vi "Clean errors.vi"(8 "error in (no error)":errorcluster) -> (0 "error out":errorcluster)   [LabVIEW 2020, in "Error Handler.lvlib"]
uses:
  Error Handler.lvlib
  Error Hander Def.ctl
  Def/Queue_Function Def.ctl
  Def/Queue_Method Def.ctl
  Def/Queue_Def.ctl
  <vilib>/MultiError/TokenizeJSON/Multi Error Cluster.lvlib
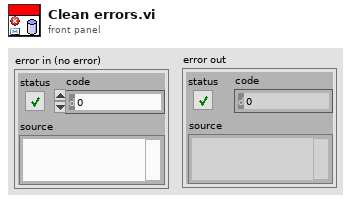
[diagram p1: front panel]
types:
  T1 = typedef "Queue_Def.ctl" = cluster{"Message":string, "Data":variant}
  T2 = typedef "Queue_Method Def.ctl" = enum16{"Initialize", "Read", "Write", "Insert", "Get_Specific_Quene_Status", "Flush Speciffic Quene", "Release All Quenes"}
  T3 = typedef "Queue_Function Def.ctl" = enum16{"MHL", "Return(Watch dog)", "Event Log", "Error Log"}
  T4 = typedef "Error Handler.lvlib/Error Hander Def.ctl" = cluster{"Time":timestamp, "Data":errorcluster}
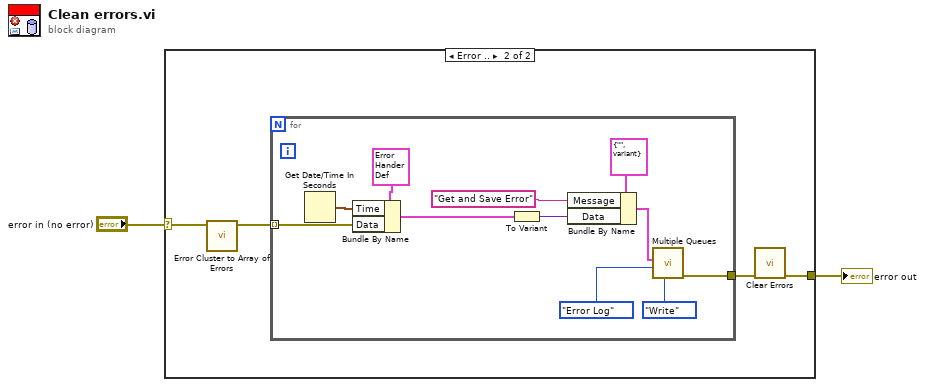
[diagram p0: block diagram]
diagram:
  n1 = case shown="Error .." "error in (no error)" {
    selector: "error in (no error)" -> [w3 w7]
    tunnel: [w3 w4] -> w1
    frame No Error {
    }
    frame Error {
      n2 = call <vilib>:"Error Cluster to Array of Errors.vi"("error"=w7) -> ("array of errors"=w6:errorcluster[])  [unwired: 10 in]
      n3 = for {
        tunnel: w6 -> [w16] mode=indexing
        tunnel: [w8] -> w5
        n4 = Get Date/Time In Seconds() -> (seconds since 1Jan1904=w17:timestamp)
        n5 = Bundle By Name(cluster=T4 {"Time"=timestamp(0 s since 1904-01-01), "Data"={"status"=FALSE, "code"=0, "source"=""}} ("Error Data"), "Time"=w17, "Data"=w16) -> (w9:T4)
        n6 = To Variant(anything=w9) -> (Variant=w15:variant)
        n7 = Bundle By Name(cluster=T1 {"Message"="", "Data"=variant} ("Quenes"), "Message"="Get and Save Error", "Data"=w15) -> (w13:T1)
        n8 = call "Multiple Queues.vi"("Method"=Queue_Method_Def."Write", "Functions"=Queue_Function_Def."Error Log", "Quenes"=w13) -> ("error out"=w8:errorcluster)  [unwired: 6 in, 2 out]
      }
      n9 = call <vilib>:"Clear Errors.vi"("error in (no error)"=w5) -> ("error out"=w4:errorcluster)  [unwired: 5 in, 1 out]
    }
  }
  "error out" <- w1
